vi "WK6440B_Test.vi"(8 "error in (no error)":errorcluster, 11 "WK6440B in":refnum<class "WK6440B.lvclass">) -> (0 "error out":errorcluster, 3 "WK6440B out":refnum<class "WK6440B.lvclass">)   [LabVIEW 2019, in "WK6440B.lvclass"]
uses:
  WK6440B.lvclass
  <vilib>/Platform/TimedLoop/XDataNode/timing_clust.ctl
  <vilib>/Platform/TimedLoop/XDataNode/nitl_modes.ctl
  <vilib>/Platform/TimedLoop/XDataNode/wakeup.ctl
  InstrumentSetup.vi
  <vilib>/platform/TimedLoop/XDataNode/XDataNode.xnode
  <vilib>/Platform/TimedLoop/XDataNode/XDNodeRunTimeDep.lvlib
  InstrControl.lvclass
panel:
  out "Resistance in MOhm":dbl
  out "Capacitance in pF":dbl
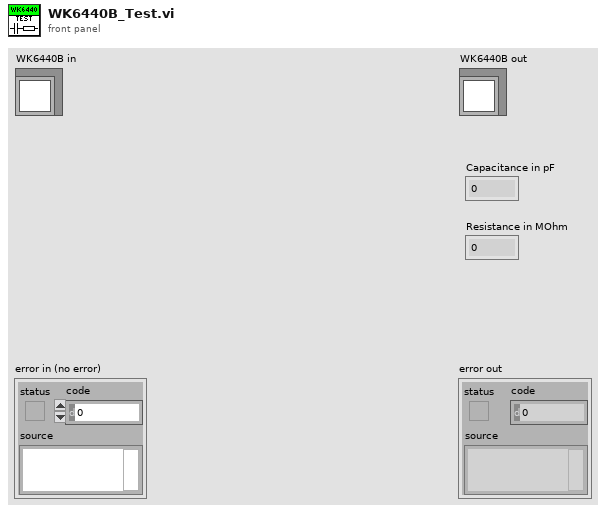
[diagram p1: front panel]
types:
  T1 = cluster{"KE 2410":cluster{"Instrument name":string, "address":refnum<visa-resource-name>, "Instrument type":u16}, "KE 6517":cluster{"Instrument name":string, "address":refnum<visa-resource-name>, "Instrument type":u16}, "KE 487":cluster{"Instrument name":string, "address":refnum<visa-resource-name>, "Instrument type":u16}, "KE 236":cluster{"Instrument name":string, "address":refnum<visa-resource-name>, "Instrument type":u16}, "WK 6440B":cluster{"Instrument name":string, "address":refnum<visa-resource-name>, "Instrument type":u16}, "WK 6425":cluster{"Instrument name":string, "address":refnum<visa-resource-name>, "Instrument type":u16}, "Pickering Matrix":cluster{"Instrument name":string, "address":refnum<visa-resource-name>, "Instrument type":u16}, "KE 2000":cluster{"Instrument name":string, "address":refnum<visa-resource-name>, "Instrument type":u16}, "KE3706A Switching":cluster{"Instrument name":string, "address":refnum<visa-resource-name>, "Instrument type":u16}, "KE 2657A":cluster{"Instrument name":string, "address":refnum<visa-resource-name>, "Instrument type":u16}, "R_METAL KE2410":cluster{"Instrument name":string, "address":refnum<visa-resource-name>, "Instrument type":u16}}
  T2 = cluster{"RC Configuration":u16, "AC amplitude [V]":dbl, "AC frequency [Hz]":i32, "WK6440B":refnum<class "WK6440B.lvclass">}
  T3 = typedef "XDNodeRunTimeDep.lvlib/timing_clust.ctl" = cluster{"Expected End [f-1]":u64, "Actual End [f-1]":u64, "Finished Late? [f-1]":bool, "Expected End [i-1]":u64, "Actual End [i-1]":u64, "Finished Late? [i-1]":bool, "Expected Start [i]":u64, "Actual Start [i]":u64, "Expected Start [f]":u64, "Actual Start [f]":u64, "Source Name":string, "Structure Name":string, "Period":i64, "Deadline":i64, "Offset":i64, "Start":i64, "Priority":i32, "Timeout":i32, "Mode":T4, "Wakeup Reason":T5, "Error":errorcluster, "Source Type":string, "Secondary Source Type":string, "Global End Time":u64, "Global Start Time":u64, "Frame Duration":u64, "Iteration Duration":u64, "Assigned CPU":i32, "I/O Scan Engine Mode":u32}
  T4 = typedef "XDNodeRunTimeDep.lvlib/nitl_modes.ctl" = enum32{"No Change", "Process missed periods, maintain original phase", "Discard missed periods, maintain original phase", "Process missed periods, ignore original phase", "Discard missed periods, ignore original phase"}
  T5 = typedef "XDNodeRunTimeDep.lvlib/wakeup.ctl" = enum32{"Normal", "Aborted", "Asynchronous wakeup", "Timing source error", "Timed loop error", "Timeout"}
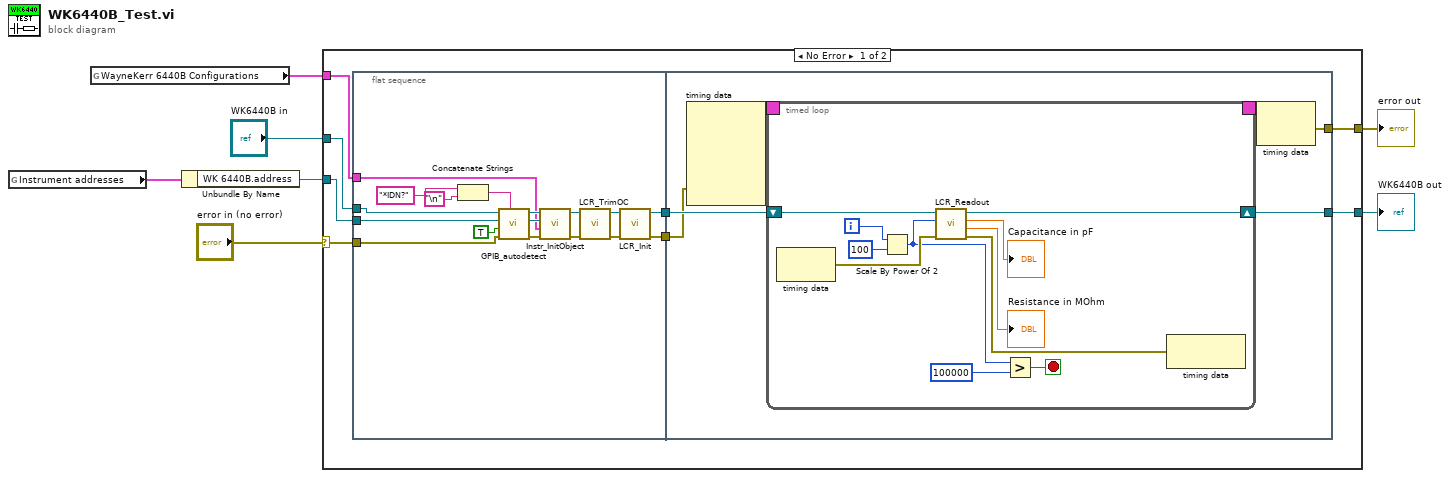
[diagram p0: block diagram]
diagram:
  n1 = global read "InstrumentSetup.vi" "Instrument addresses"() -> (w2:T1)
  n2 = global read "InstrumentSetup.vi" "WayneKerr 6440B Configurations"() -> (w3:T2)
  n3 = Unbundle By Name(w2) -> ("WK 6440B.address"=w1:refnum<visa-resource-name>)
  n4 = case shown="No Error" "error in (no error)" {
    selector: "error in (no error)" -> [w10 w61]
    tunnel: [w15 w61] -> w6
    tunnel: [w14 w60] -> w4
    tunnel: "WK6440B in" -> [w11 w60]
    tunnel: w3 -> [w9 _]
    tunnel: w1 -> [w8 _]
    frame No Error {
      n5 = flat-sequence {
        tunnel: w11 -> [w28]
        tunnel: w10 -> [w24]
        tunnel: [w30] -> w13
        tunnel: [w29] -> w12
        tunnel: w9 -> [w21]
        tunnel: w8 -> [w20]
        tunnel: w13 -> [w35]
        tunnel: w12 -> [w33]
        tunnel: [w36] -> w15
        tunnel: [w34] -> w14
        frame #0 {
          n6 = Concatenate Strings("*IDN?" ("regular expression"), "\n") -> (w16:string)
          n7 = call-dynamic "GPIB_autodetect.vi"("ID command"=w16, "error in (no error)"=w24, "Verify GPIB address"=TRUE, "Instrument address in"=w20, "InstrControl in"=w28) -> ("error out"=w26:errorcluster, "Instrument address out"=w25:refnum<visa-resource-name>, "InstrControl out"=w27:refnum<class "WK6440B.lvclass">)  [unwired: 4 in]
          n8 = call-dynamic "Instr_InitObject.vi"("error in (no error)"=w26, "Instrument Configuration"=w21, "Instrument address"=w25, "WK6440B in"=w27) -> ("error out"=w23:errorcluster, "WK6440B out"=w22:refnum<class "WK6440B.lvclass">)  [unwired: 6 in]
          n9 = call-dynamic "LCR_TrimOC.vi"("error in (no error)"=w23, "LCRControl in"=w22) -> ("error out"=w31:errorcluster, "LCRControl out"=w32:refnum<class "WK6440B.lvclass">)  [unwired: 8 in]
          n10 = call-dynamic "LCR_Init.vi"("error in (no error)"=w31, "LCRControl in"=w32) -> ("error out"=w29:errorcluster, "LCRControl out"=w30:refnum<class "WK6440B.lvclass">)  [unwired: 8 in]
        }
        frame #1 {
          n11 = node-c288(w33) -> (w38:T3)  [unwired: 4 in]
          n12 = timed-loop {
            timing: w38 -> [_]
            timing-out: [_] -> w37
            shift-right: [w41] -> w34
            shift-left: w35 -> [w42]
            i -> [w44]
            stop <- w46 stop-if-true
            n13 = node-c288() -> (w49:errorcluster)  [unwired: 1 in]
            n14 = Scale By Power Of 2(n=w44, x=100) -> (x*2^n=w43:i32)
            n15 = call-dynamic "LCR_Readout.vi"("error in (no error)"=w49, "Frequency in Hz"=w43, "WK6440B in"=w42) -> ("error out"=w48:errorcluster, "Resistance in Ohm"=→"Resistance in MOhm":dbl, "Capacitance in pF"=→"Capacitance in pF":dbl, "WK6440B out"=w41:refnum<class "WK6440B.lvclass">)  [unwired: 5 in]
            n16 = Greater?(x=w43, y=100000) -> (0:w46:bool)
            n17 = node-c288(w48) -> ()  [unwired: 1 out]
          }
          n18 = node-c288(w37) -> (w36:errorcluster)
        }
      }
    }
    frame Error {
    }
  }
  "error out" <- w6
  "WK6440B out" <- w4
